vi "GetSerializableData.vi"(8 "error in (no error)":errorcluster, 9 "Options":T1, 10 "Data in":T3, 11 "BlueSerializable in":refnum<class "BlueSerializable.lvclass">) -> (0 "error out":errorcluster, 2 "Data out":T3, 3 "BlueSerializable out":refnum<class "BlueSerializable.lvclass">)   [LabVIEW 2020, in "BlueSerialization.lvlib" / "BlueSerializable.lvclass"]
doc: "Dynamic Dispatch VI which returns a variant of an entire inheritance heirarchy's serializable data which can later be serialized by a <b>SerializerBase</b> into any format."
uses:
  BlueSerializable.lvclass
  BlueSerializer/Support/GetSerializableDataCluster.ctl
  BlueSerializer/GetSerializableDataAction.ctl
  BlueSerializer/Support/GetSerializableDataClusterClass.ctl
  BlueSerializer/Support/SerializableDataGetDataAction.ctl
  BlueSerializer/ClassNameAndVersion.ctl
  <vilib>/Utility/EditLVLibs/LibVersion.ctl
  BlueSerializer/SerializeOptionsPayload.ctl
  BlueSerializer/SerializeOptions.ctl
  BlueSerializer/ClassNameCacheMap.ctl
  BlueSerializer/ClassNameObj.ctl
  BlueSerializable.lvclass/BlueSerializable.ctl
  BlueSerializer/BlueSerializer.lvclass
  <vilib>/Utility/EditLVLibs/Edit LVLibs.lvlib
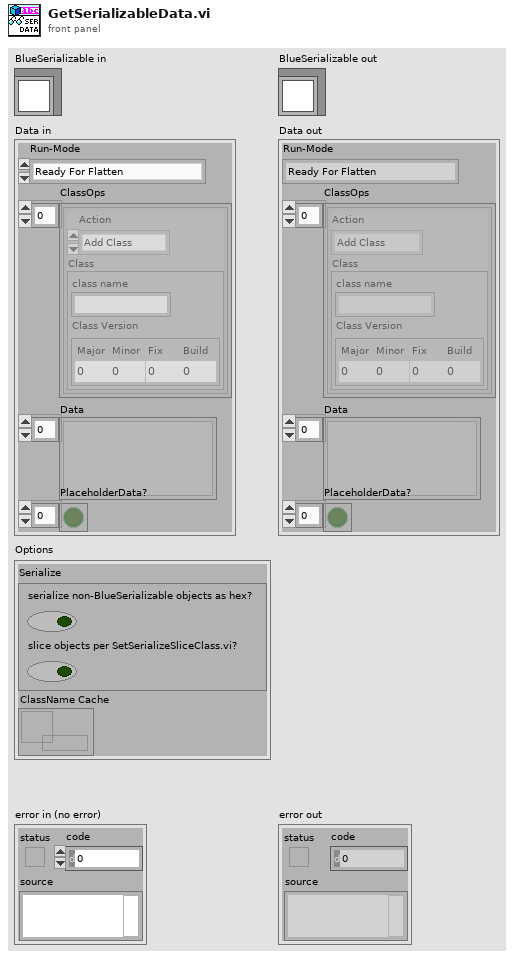
[diagram p1: front panel]
types:
  T1 = typedef "BlueSerialization.lvlib/BlueSerializer.lvclass/SerializeOptionsPayload.ctl" = cluster{"Serialize":T2, "ClassName Cache":refnum<data-value>}
  T2 = typedef "BlueSerialization.lvlib/BlueSerializer.lvclass/SerializeOptions.ctl" = cluster{"serialize non-BlueSerializable objects as hex?":bool, "slice objects per SetSerializeSliceClass.vi?":bool}
  T3 = typedef "BlueSerialization.lvlib/BlueSerializer.lvclass/GetSerializableDataCluster.ctl" = cluster{"Run-Mode":T4, "ClassOps":T5[], "Data":variant[], "PlaceholderData?":bool[]}
  T4 = typedef "BlueSerialization.lvlib/BlueSerializer.lvclass/GetSerializableDataAction.ctl" = enum16{"Ready For Flatten", "Unmodified Data Access"}
  T5 = typedef "BlueSerialization.lvlib/BlueSerializer.lvclass/GetSerializableDataClusterClass.ctl" = cluster{"Action":T6, "Class":T7}
  T6 = typedef "BlueSerialization.lvlib/BlueSerializer.lvclass/SerializableDataGetDataAction.ctl" = enum16{"Add Class", "Drop Class"}
  T7 = typedef "BlueSerialization.lvlib/BlueSerializer.lvclass/ClassNameAndVersion.ctl" = cluster{"class name":string, "Class Version":T8}
  T8 = typedef "Edit LVLibs.lvlib/LibVersion.ctl" = cluster{"Major":u16, "Minor":u16, "Fix":u16, "Build":u16}
  T9 = typedef "BlueSerialization.lvlib/BlueSerializable.lvclass/SerializableData.ctl" = cluster{"LibVersion":u8}
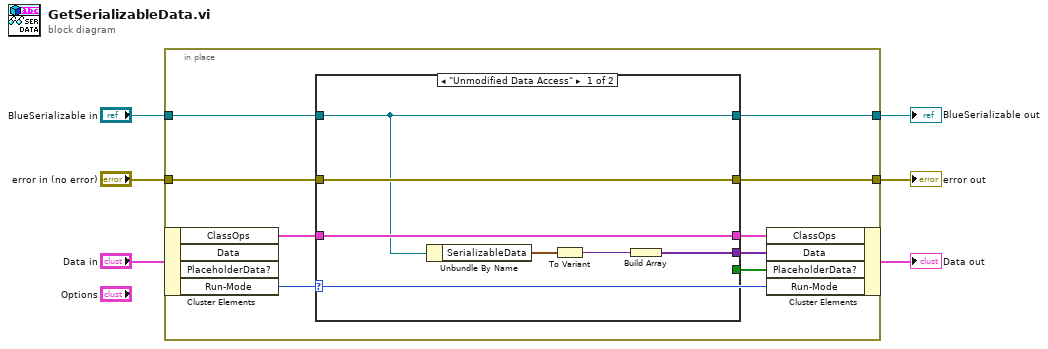
[diagram p0: block diagram]
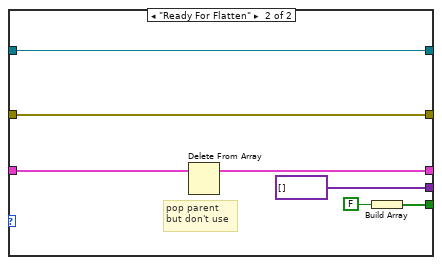
[diagram p2: hidden frame]
diagram:
  n1 = in-place {
    in-place-border: "BlueSerializable in" -> [w9]
    in-place-border: [w8] -> w4
    in-place-border: "error in (no error)" -> [w11]
    in-place-border: [w13] -> w2
    n2 = in-place-cluster #1("Data in") -> ("ClassOps"=w15:T5[], "Run-Mode"=w10:T4)  [unwired: 2 out]
    n3 = case shown="\"Unmodified Data Access\"" w10 {
      tunnel: w15 -> [w19 w28]
      tunnel: [w19 w27] -> w14
      tunnel: [w21 w26] -> w13
      tunnel: [w20 variant[] []] -> w12
      tunnel: w11 -> [w21 w26]
      tunnel: w9 -> [w17 w25]
      tunnel: [w17 w25] -> w8
      tunnel: [_ w22] -> w7
      frame "Unmodified Data Access" {
        n4 = Unbundle By Name(w17) -> ("SerializableData"=w18:T9)
        n5 = To Variant(anything=w18) -> (Variant=w16:variant)
        n6 = Build Array(w16) -> (w20:variant[])
      }
      frame "Ready For Flatten" {
        # "pop parent\nbut don't use"
        n7 = Delete From Array(array=w28) -> (array with subset deleted=w27:T5[])  [unwired: 2 in, 1 out]
        n8 = Build Array(FALSE) -> (w22:bool[])
      }
    }
    n9 = in-place-cluster #1("ClassOps"=w14, "Data"=w12, "PlaceholderData?"=w7, "Run-Mode"=w10) -> (→"Data out":T3)
  }
  "error out" <- w2
  "BlueSerializable out" <- w4
